vi "AE - Bluetooth ButtonAccData.vi"(8 "error in (no error)":errorcluster, 11 "Wiimote":i32) -> (0 "error out":errorcluster, 3 "Wiimote State":T1)   [LabVIEW 2010]
uses:
  AE Cores/Custom Controls/WiimoteState.ctl
  AE Cores/AE - Bluetooth Enum.ctl
panel:
  # "Accelerometers"
  # "Buttons"
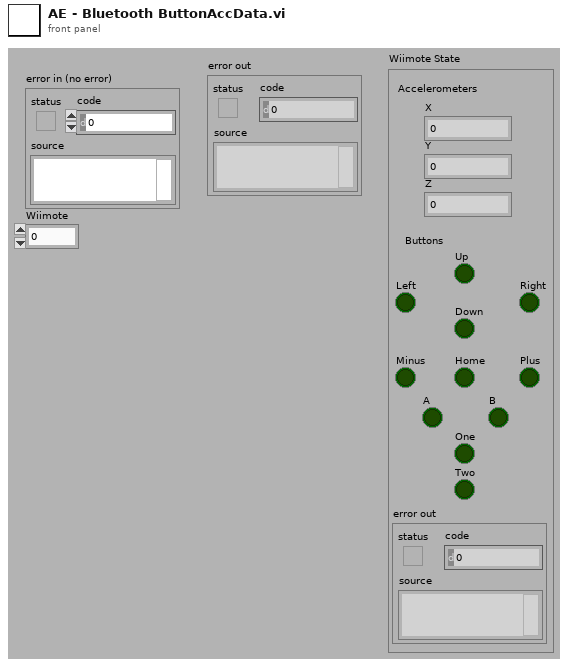
[diagram p1: front panel]
types:
  T1 = typedef "WiimoteState.ctl" = cluster{"X":sgl, "Y":sgl, "Z":sgl, "A":bool, "B":bool, "Down":bool, "Home":bool, "Left":bool, "Minus":bool, "One":bool, "Plus":bool, "Right":bool, "Two":bool, "Up":bool, "error out":errorcluster}
  T2 = typedef "AE - Bluetooth Enum.ctl" = enum16{"Initialise", "Pair All Wiimotes", "Connect All Wiimotes", "Set Rumble", "Set LED", "Get Button + Acc Data", "Get IR Data", "Get Battery", "Get Wiimote Reference", "Reorder Wiimotes", "devReport"}
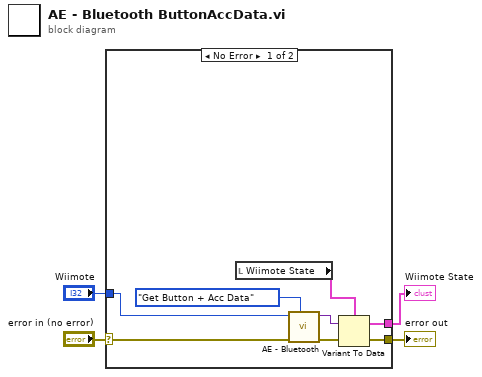
[diagram p0: block diagram]
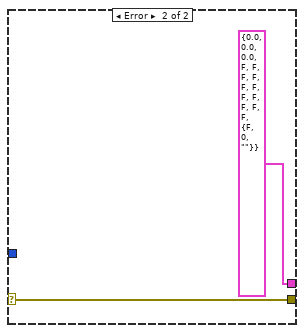
[diagram p2: hidden frame]
diagram:
  n1 = case shown="No Error" "error in (no error)" {
    selector: "error in (no error)" -> [w11 w14]
    tunnel: [w8 w14] -> w3
    tunnel: [w6 T1 {"X"=0.0, "Y"=0.0, "Z"=0.0, "A"=FALSE, "B"=FALSE, "Down"=FALSE, "Home"=FALSE, "Left"=FALSE, "Minus"=FALSE, "One"=FALSE, "Plus"=FALSE, "Right"=FALSE, "Two"=FALSE, "Up"=FALSE, "error out"={"status"=FALSE, "code"=0, "source"=""}} ("Wiimote State")] -> w2
    tunnel: "Wiimote" -> [w5 _]
    frame No Error {
      n2 = local read "Wiimote State"() -> (w7:T1)
      n3 = call "AE - Bluetooth.vi"("Enum"=AE_-_Bluetooth_Enum."Get Button + Acc Data", "error in (no error)"=w11, "Variant In"=w5) -> ("error out"=w9:errorcluster, "Variant Out"=w10:variant)  [unwired: 6 in, 1 out]
      n4 = Variant To Data(error in=w9, Variant=w10, type=w7) -> (error out=w8:errorcluster, data=w6:T1)
    }
    frame Error {
    }
  }
  "error out" <- w3
  "Wiimote State" <- w2
